vi "CreateDataStructures.vi"(8 "Error In":errorcluster) -> (0 "Error Out":errorcluster, 3 "Data Structures":T1)   [LabVIEW 2012]
uses:
  DataStructures.ctl
  HardwareDisplayData.ctl
  HardwareLogData.ctl
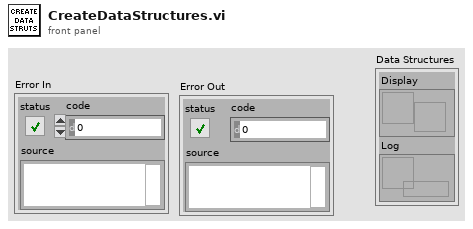
[diagram p1: front panel]
types:
  T1 = typedef "DataStructures.ctl" = cluster{"Display":refnum<notifier>, "Log":refnum<queue>}
  T2 = typedef "HardwareLogData.ctl" = cluster{"Timestamp":timestamp, "Data":T3}
  T3 = typedef "HardwareDisplayData.ctl" = cluster{"Heater":dbl, "MFC":dbl}
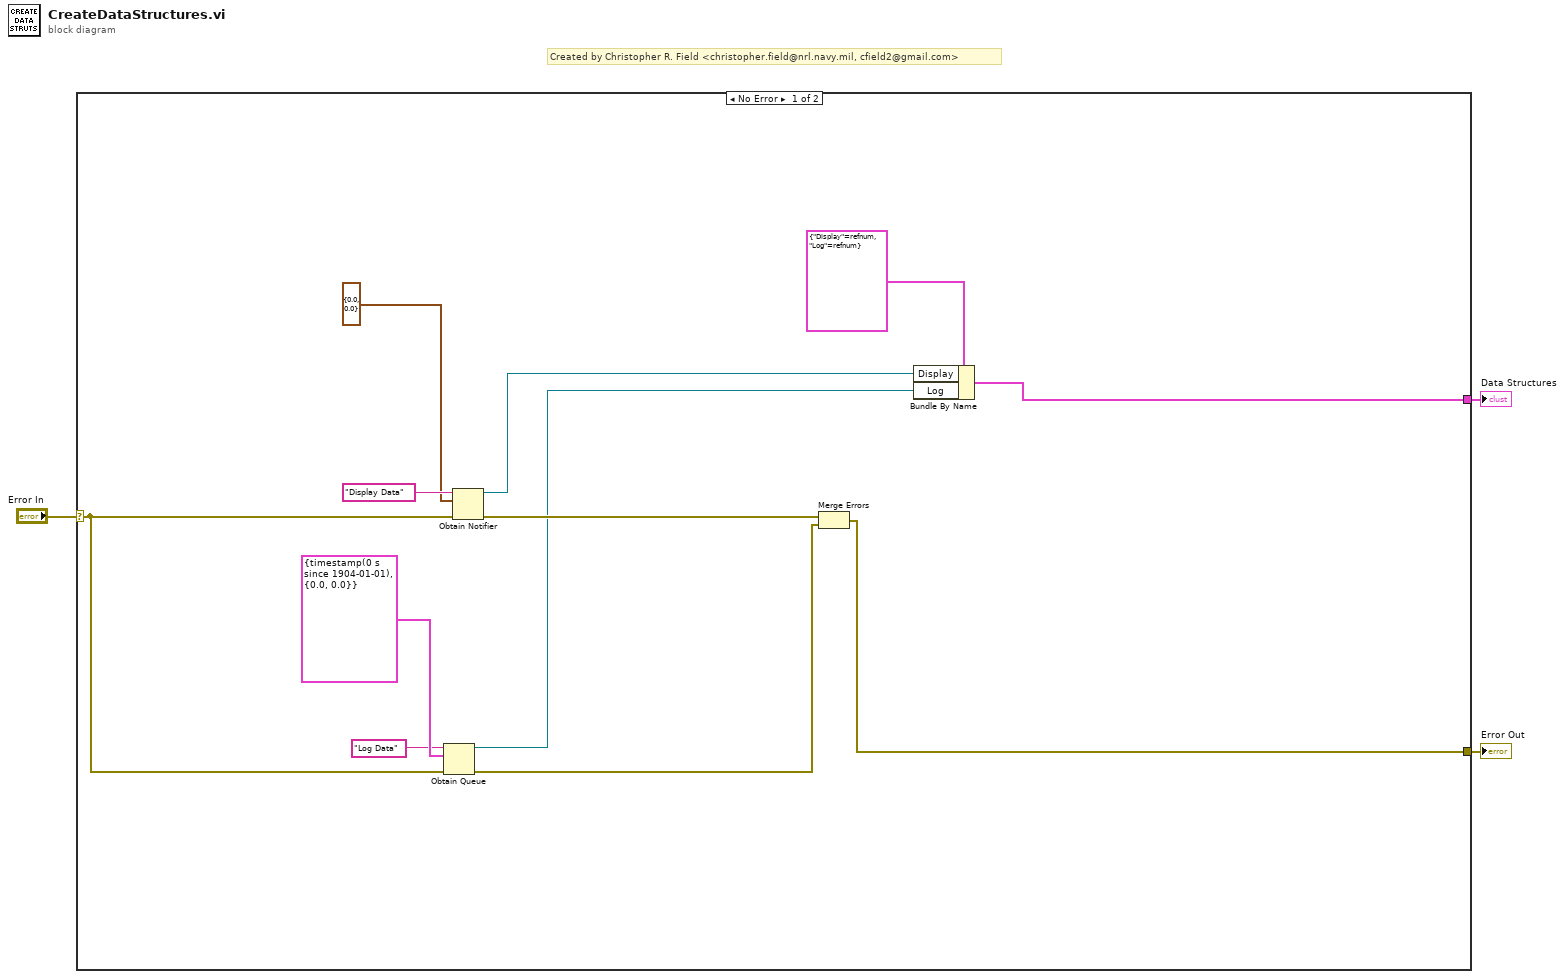
[diagram p0: block diagram]
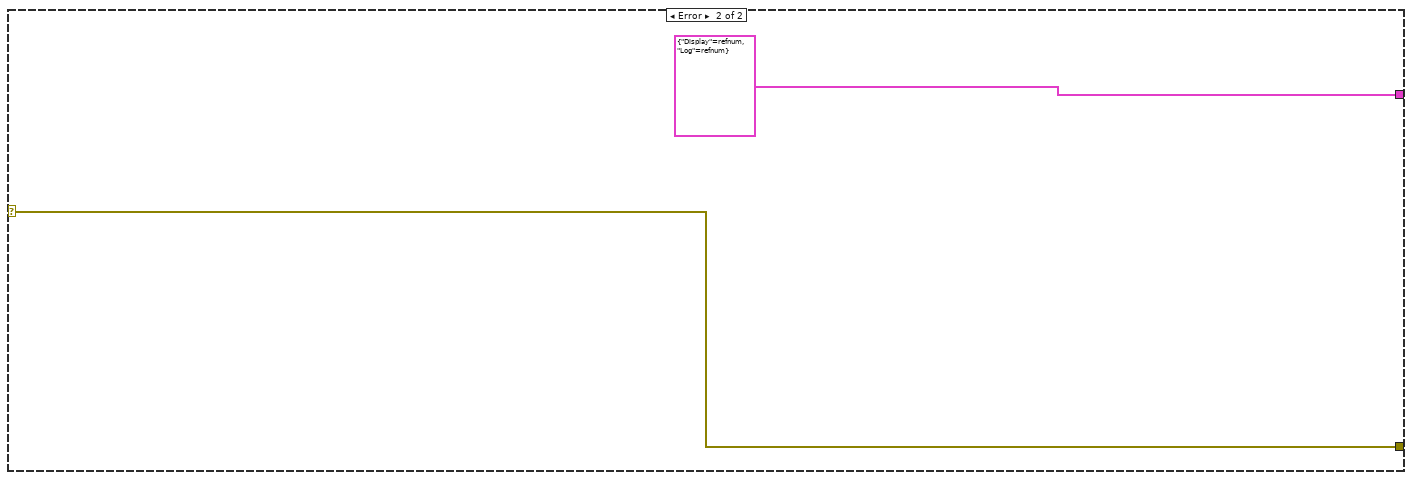
[diagram p2: hidden frame]
diagram:
  # "Created by Christopher R. Field <christopher.field@nrl.navy.mil, cfield2@gmail.com>"
  n1 = case shown="No Error" "Error In" {
    selector: "Error In" -> [w9 w17]
    tunnel: [w13 w17] -> w2
    tunnel: [w4 T1 {"Display"=refnum, "Log"=refnum} ("Data Structures")] -> w1
    frame No Error {
      n2 = Obtain Queue(name (unnamed)="Log Data", element data type=T2 {"Timestamp"=timestamp(0 s since 1904-01-01), "Data"={"Heater"=0.0, "MFC"=0.0}} ("Hardware Log Data"), error in (no error)=w9) -> (queue out=w5:refnum<queue>, error out=w8:errorcluster)  [unwired: 2 in, 1 out]
      n3 = Obtain Notifier(name (unnamed)="Display Data", notification data type=T3 {"Heater"=0.0, "MFC"=0.0} ("Hardware Display Data"), error in (no error)=w9) -> (notifier out=w6:refnum<notifier>, error out=w14:errorcluster)  [unwired: 1 in, 1 out]
      n4 = Merge Errors(w14, w8) -> (w13:errorcluster)
      n5 = Bundle By Name(cluster=T1 {"Display"=refnum, "Log"=refnum} ("Data Structures"), "Display"=w6, "Log"=w5) -> (w4:T1)
    }
    frame Error {
    }
  }
  "Error Out" <- w2
  "Data Structures" <- w1
